vi "ITX to LV 2.1.vi"(8 "error in":errorcluster, 11 "file (use dialog)":path=path "P:/sample/GaAs/GaAs quantum dots/2008/PL Map/A1 735/060731ASBA_A1_6.0.itx") -> (0 "error out":errorcluster, 1 "1D Arrays":cluster{"key":string, "1D Array":dbl[]}[](array[cluster]), 2 "Notes":string, 3 "Data (Dictionary)":T1[](array[typedef]), 4 "Commands":string, 6 "2D Arrays":cluster{"key":string, "2D Array":dbl[][]}[](array[cluster]))   [LabVIEW 2016, in "LV to ITX.lvclass"]
uses:
  LV to ITX.lvclass
  Typedefs/Dictionary--cluster.ctl
  <userlib>/_OpenG.lib/string/string.llb/Trim Whitespace (String)__ogtk.vi
panel:
  out "parse 2 (ms)":u32
  out "parse 2":u32
  out "parse 1 (ms)":u32
  out "open file (ms)":u32
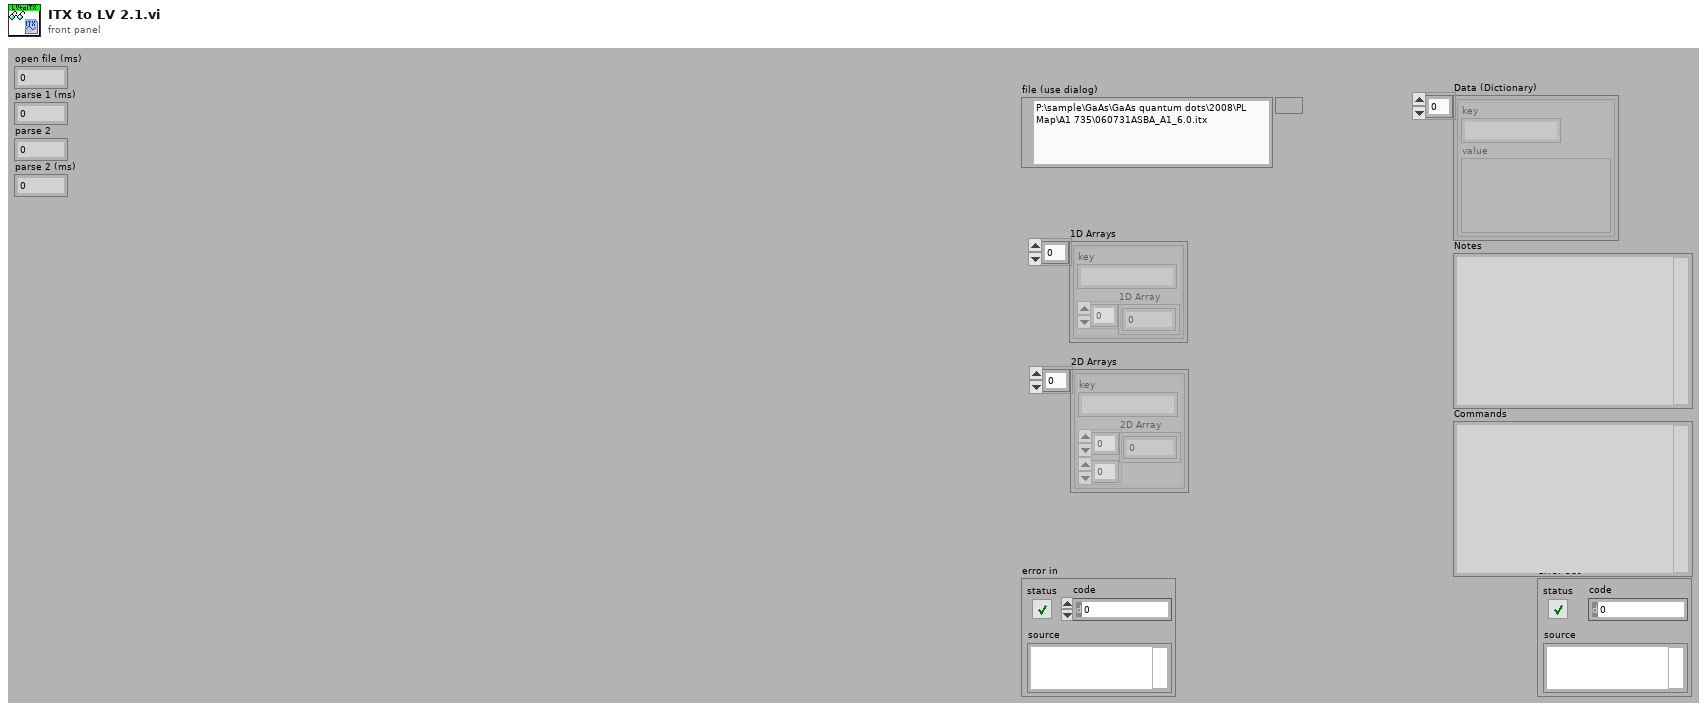
[diagram p1: front panel]
types:
  T1 = typedef "LV to ITX.lvclass/Dictionary--cluster.ctl" = cluster{"key":string, "value":variant}
  T2 = cluster{"result string":string, "1D Array":dbl[]}
  T3 = cluster{"result string":string, "2D Array":dbl[][]}
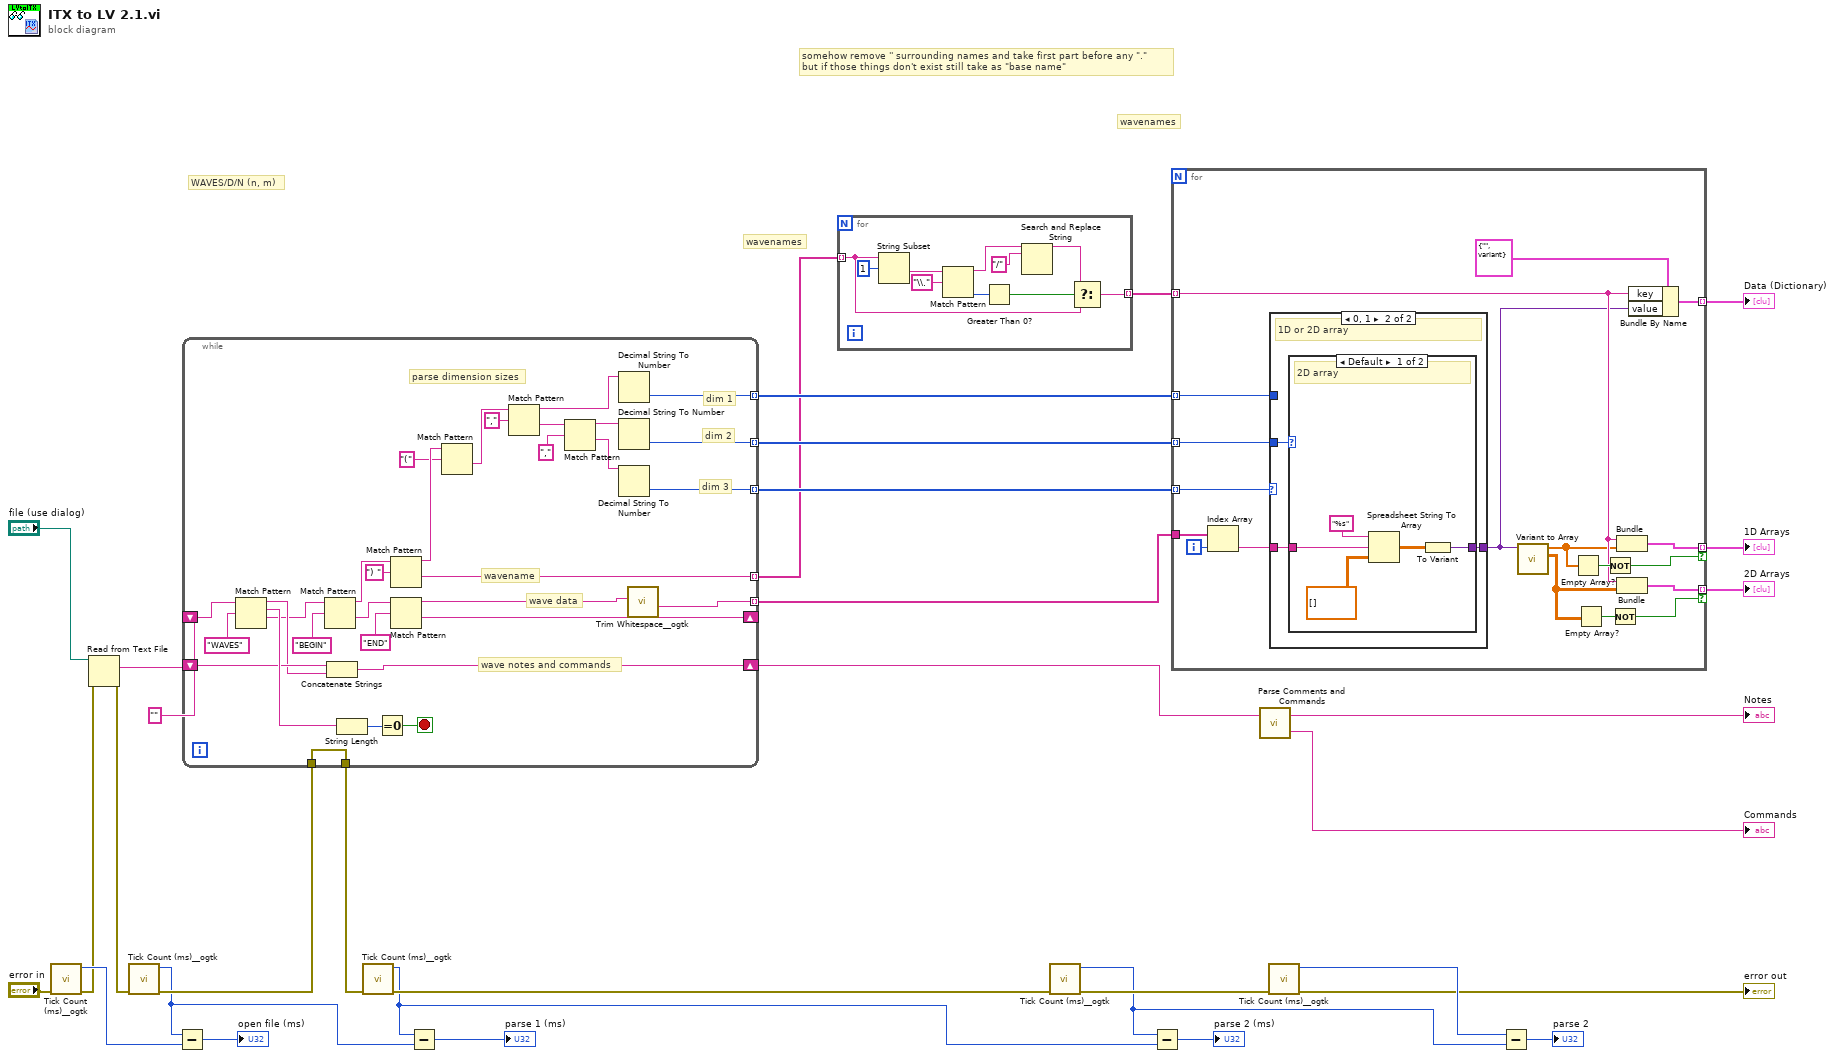
[diagram p0: block diagram]
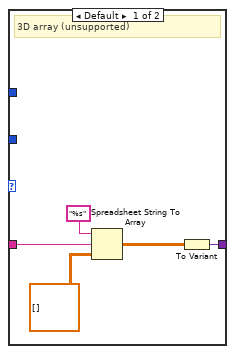
[diagram p2: hidden frame]
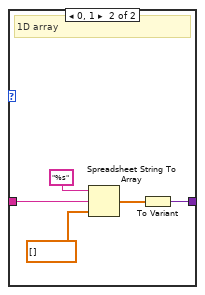
[diagram p3: hidden frame]
diagram:
  # "wavenames"
  # "wavenames"
  # "somehow remove '' surrounding names and take first part before any \".\"\nbut if those things don't exist still take as \"base name\""
  # "WAVES/D/N (n, m)"
  n1 = call <userlib>:"Tick Count (ms)__ogtk.vi"("error in (no error)"="error in") -> ("error out"=w27:errorcluster, "millisecond timer value"=w29:u32)  [unwired: 9 in]
  n2 = Read from Text File(file (use dialog)="file (use dialog)", error in=w27) -> (text=w16:string, error out=w26:errorcluster)  [unwired: 1 in, 3 out]
  n3 = call <userlib>:"Tick Count (ms)__ogtk.vi"("error in (no error)"=w26) -> ("error out"=w24:errorcluster, "millisecond timer value"=w8:u32)  [unwired: 9 in]
  n4 = Subtract(x=w8, y=w29) -> (x-y=→"open file (ms)":u32)
  n5 = while {
    tunnel: [w38] -> w4 mode=indexing
    shift-right: [w62] -> _
    shift-left: w16 -> [w50]
    tunnel: [w58] -> w10 mode=indexing
    shift-right: [w53] -> w3
    shift-left: "" ("regular expression") -> [w52]
    tunnel: [w48] -> w25
    tunnel: w24 -> [w48]
    tunnel: [w40] -> w14 mode=indexing
    tunnel: [w42] -> w13 mode=indexing
    tunnel: [w33] -> w11 mode=indexing
    stop <- w59 stop-if-true
    # "dim 3"
    # "dim 2"
    # "dim 1"
    # "wave data"
    # "wave notes and commands"
    # "parse dimension sizes"
    # "wavename"
    n6 = Match Pattern(string=w50, regular expression="WAVES") -> (before substring=w51:string, match substring=w61:string, after substring=w47:string)  [unwired: 2 out]
    n7 = Match Pattern(string=w47, regular expression="BEGIN" ("regular expression 2")) -> (before substring=w49:string, after substring=w63:string)  [unwired: 3 out]
    n8 = Concatenate Strings(w52, w51) -> (w53:string)
    n9 = String Length(string=w61) -> (length=w60:i32)
    n10 = Equal To 0?(x=w60) -> (x = 0?=w59:bool)
    n11 = Match Pattern(string=w49, regular expression=") ") -> (before substring=w46:string, after substring=w58:string)  [unwired: 3 out]
    n12 = Match Pattern(string=w63, regular expression="END" ("regular expression 3")) -> (before substring=w39:string, after substring=w62:string)  [unwired: 3 out]
    n13 = Match Pattern(string=w46, regular expression="(") -> (after substring=w44:string)  [unwired: 4 out]
    n14 = Match Pattern(string=w44, regular expression=",") -> (before substring=w41:string, after substring=w37:string)  [unwired: 3 out]
    n15 = Match Pattern(string=w37, regular expression=",") -> (before substring=w35:string, after substring=w36:string)  [unwired: 3 out]
    n16 = Decimal String To Number(string=w41) -> (number=w40:i32)  [unwired: 2 in, 1 out]
    n17 = Decimal String To Number(string=w35) -> (number=w42:i32)  [unwired: 2 in, 1 out]
    n18 = Decimal String To Number(string=w36) -> (number=w33:i32)  [unwired: 2 in, 1 out]
    n19 = call-poly <userlib>:"Trim Whitespace__ogtk.vi"("String in"=w39) -> ("String out"=w38:string)  [unwired: 6 in]
  }
  n20 = call <userlib>:"Tick Count (ms)__ogtk.vi"("error in (no error)"=w25) -> ("error out"=w15:errorcluster, "millisecond timer value"=w7:u32)  [unwired: 9 in]
  n21 = Subtract(x=w7, y=w8) -> (x-y=→"parse 1 (ms)":u32)
  n22 = for {
    tunnel: w10 -> [w65] mode=indexing
    tunnel: [w66] -> w5 mode=indexing
    n23 = String Subset(string=w65, offset (0)=1) -> (substring=w72:string)  [unwired: 1 in]
    n24 = Match Pattern(string=w72, regular expression="\\.") -> (before substring=w68:string, offset past match=w70:i32)  [unwired: 1 in, 2 out]
    n25 = Greater Than 0?(x=w70) -> (x > 0?=w67:bool)
    n26 = Search and Replace String(input string=w68, search string="/") -> (result string=w64:string)  [unwired: 6 in, 3 out]
    n27 = Select(t=w64, s=w67, f=w65) -> (s? t:f=w66:string)
  }
  n28 = call <userlib>:"Tick Count (ms)__ogtk.vi"("error in (no error)"=w15) -> ("error out"=w21:errorcluster, "millisecond timer value"=w6:u32)  [unwired: 9 in]
  n29 = Subtract(x=w6, y=w7) -> (x-y=→"parse 2 (ms)":u32)
  n30 = for {
    tunnel: w4 -> [w91]
    tunnel: w5 -> [w76] mode=indexing
    tunnel: [w89] -> w12 mode=indexing
    tunnel: w14 -> [w86] mode=indexing
    tunnel: w13 -> [w85] mode=indexing
    tunnel: w11 -> [w87] mode=indexing
    tunnel: [w83] -> w2 mode=indexing if=w78
    tunnel: [w82] -> w1 mode=indexing if=w77
    i -> [w90]
    n31 = Index Array(array=w91, index=w90) -> (element=w84:string)
    n32 = case shown="0, 1" w87 {
      tunnel: w84 -> [w94 w98]
      tunnel: [w96 w99] -> w75
      tunnel: w86 -> [_ _]
      tunnel: w85 -> [_ w97]
      frame Default {
        # "3D array (unsupported)"
        n33 = Spreadsheet String To Array(format string="%s", spreadsheet string=w94, array type (2D Dbl)=dbl[][][] []) -> (array=w93:dbl[][][])  [unwired: 1 out]
        n34 = To Variant(anything=w93) -> (Variant=w96:variant)
      }
      frame 0, 1 {
        # "1D or 2D array"
        n35 = case shown="Default" w97 {
          tunnel: [w104 w109] -> w99
          tunnel: w98 -> [w102 w107]
          frame Default {
            # "2D array"
            n36 = Spreadsheet String To Array(format string="%s", spreadsheet string=w102, array type (2D Dbl)=dbl[][] []) -> (array=w101:dbl[][])  [unwired: 1 out]
            n37 = To Variant(anything=w101) -> (Variant=w104:variant)
          }
          frame 0, 1 {
            # "1D array"
            n38 = Spreadsheet String To Array(format string="%s", spreadsheet string=w107, array type (2D Dbl)=dbl[] []) -> (array=w106:dbl[])  [unwired: 1 out]
            n39 = To Variant(anything=w106) -> (Variant=w109:variant)
          }
        }
      }
    }
    n40 = call "Variant to Array.vi"("value"=w75) -> ("2D Array"=w80:dbl[][], "1D Array"=w74:dbl[])  [unwired: 8 in, 1 out]
    n41 = Empty Array?(array=w74) -> (empty?=w81:bool)
    n42 = Empty Array?(array=w80) -> (empty?=w79:bool)
    n43 = Not(x=w81) -> (.not. x?=w78:bool)
    n44 = Not(x=w79) -> (.not. x?=w77:bool)
    n45 = Bundle("result string"=w76, "1D Array"=w74) -> (w83:T2)  [unwired: 1 in]
    n46 = Bundle("result string"=w76, "2D Array"=w80) -> (w82:T3)  [unwired: 1 in]
    n47 = Bundle By Name(cluster=T1 {"key"="", "value"=variant} ("key-value"), "key"=w76, "value"=w75) -> (w89:T1)
  }
  "Data (Dictionary)" <- w12
  "1D Arrays" <- w2
  "2D Arrays" <- w1
  n48 = call "Parse Comments and Commands.vi"("ITX Notes and Commands"=w3) -> ("Commands"=→"Commands":string, "Notes"=→"Notes":string)  [unwired: 1 in]
  n49 = call <userlib>:"Tick Count (ms)__ogtk.vi"("error in (no error)"=w21) -> ("error out"=→"error out":errorcluster, "millisecond timer value"=w20:u32)  [unwired: 9 in]
  n50 = Subtract(x=w20, y=w6) -> (x-y=→"parse 2":u32)
